vi "plot_line_array2cluster.vi"(10 "End Point array":dbl[](array[numeric]), 11 "Start Point array":dbl[](array[numeric])) -> (2 "End Point out":cluster{"X":i32, "Y":i32}, 3 "Start Point out":cluster{"X":i32, "Y":i32})   [LabVIEW 2017]
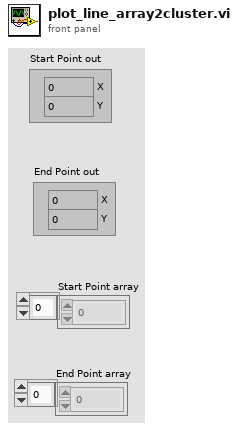
[diagram p1: front panel]
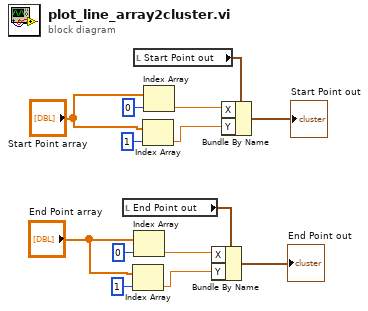
[diagram p0: block diagram]
diagram:
  n1 = local read "End Point out"() -> (w2:cluster{"X":i32, "Y":i32})
  n2 = Index Array(array="End Point array", index=1) -> (element=w9:dbl)
  n3 = local read "Start Point out"() -> (w4:cluster{"X":i32, "Y":i32})
  n4 = Index Array(array="End Point array", index=0) -> (element=w7:dbl)
  n5 = Index Array(array="Start Point array", index=1) -> (element=w11:dbl)
  n6 = Index Array(array="Start Point array", index=0) -> (element=w13:dbl)
  n7 = Bundle By Name(cluster=w2, "X"=w7, "Y"=w9) -> (→"End Point out":cluster{"X":i32, "Y":i32})
  n8 = Bundle By Name(cluster=w4, "X"=w13, "Y"=w11) -> (→"Start Point out":cluster{"X":i32, "Y":i32})
